vi "New Off Wire Message.vi"(1 "Valid":bool=TRUE, 2 "message":string, 3 "type":string) -> (0 "Off Wire Message":T1)   [LabVIEW 2016]
uses:
  Off Wire Message.ctl
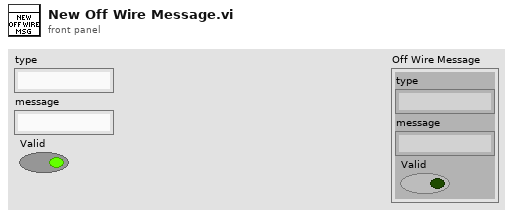
[diagram p1: front panel]
types:
  T1 = typedef "Off Wire Message.ctl" = cluster{"type":string, "message":string, "Valid":bool}
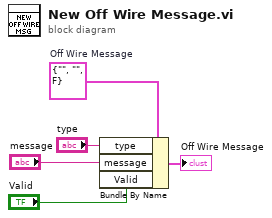
[diagram p0: block diagram]
diagram:
  w5 = T1 {"type"="", "message"="", "Valid"=FALSE}  # Off Wire Message
  n1 = Bundle By Name(cluster=w5, "type"="type", "message"="message", "Valid"="Valid") -> (→"Off Wire Message":T1)
